vi "Unload Plugin.vi"(8 "error in (no error)":errorcluster, 10 "Unique Name":string, 11 "Launcher in":refnum<class "Plugin Manager.lvclass">) -> (0 "error out":errorcluster, 3 "Launcher out":refnum<class "Plugin Manager.lvclass">)   [LabVIEW 2021, in "Plugin Manager.lvclass"]
uses:
  Plugin Manager.lvclass
  Plugin Manager.lvclass/Plugin Manager.ctl
  CIFCore/Common/Typedef/Errors.ctl
  CIFCore/Common/Utilities/Append Error Location.vi
  CIFCore/Common/CIFCoreCommon.lvlib
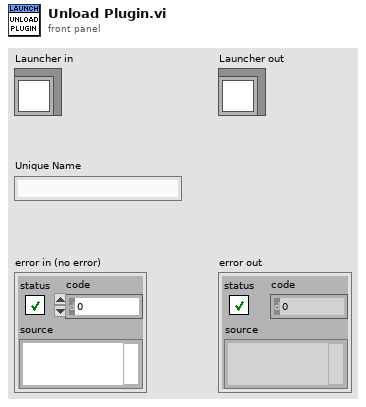
[diagram p1: front panel]
types:
  T1 = typedef "CIFCoreCommon.lvlib/Errors.ctl" = enum16{"Invalid Clock ID", "Long Sleep", "gRPC Server Not Found", "Config Parse", "Timestamp Wrap", "Delayed Execution", "Duplicate Channel", "Missing Channel", "Incorrect Type", "Flatten Error", "Unflatten Data", "Unique Name", "Plugin Not Found"}
  T2 = typedef "Plugin Manager.lvclass/Plugin Management Data.ctl" = cluster{"vi reference":refnum<vi>, "Plugin Type":string, "Unique Name":string, "Load Timestamp":u64, "gRPC Port":i32, "Version":T3}
  T3 = typedef "CIFCoreCommon.lvlib/Version.ctl" = cluster{"Major":i32, "Minor":i32, "Fix":i32, "Build":i32}
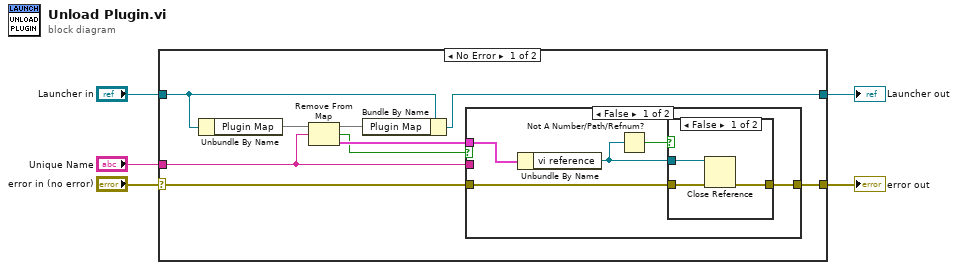
[diagram p0: block diagram]
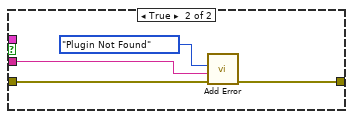
[diagram p3: hidden frame]
diagram:
  n1 = case shown="No Error" "error in (no error)" {
    selector: "error in (no error)" -> [w14 w29]
    tunnel: [w13 w29] -> w4
    tunnel: [w6 w28] -> w2
    tunnel: "Launcher in" -> [w8 w28]
    tunnel: "Unique Name" -> [w11 _]
    frame No Error {
      n2 = Unbundle By Name(w8) -> ("Plugin Map"=w12:map{string, T2})
      n3 = Remove From Map(10:w11, 11:w12) -> (1:w10:T2, 2:w9:bool, 3:w7:map{string, T2})
      n4 = Bundle By Name(cluster=w8, "Plugin Map"=w7) -> (w6:refnum<class "Plugin Manager.lvclass">)
      n5 = case shown="False" w9 {
        tunnel: w14 -> [w16 w27]
        tunnel: [w15 w24] -> w13
        tunnel: w11 -> [_ w25]
        tunnel: w10 -> [w19 _]
        frame False {
          n6 = Unbundle By Name(w19) -> ("vi reference"=w18:refnum<vi>)
          n7 = Not A Number/Path/Refnum?(number/path/refnum=w18) -> (NaN/Path/Refnum?=w17:bool)
          n8 = case shown="False" w17 {
            tunnel: w18 -> [w22 _]
            tunnel: w16 -> [w21 w23]
            tunnel: [w20 w23] -> w15
            frame False {
              n9 = Close Reference(reference=w22, error in (no error)=w21) -> (error out=w20:errorcluster)
            }
            frame True {
            }
          }
        }
        frame True {
          n10 = call "Add Error.vi"("error in (no error)"=w27, "String to Append"=w25, "Error"=Errors."Plugin Not Found") -> ("error out"=w24:errorcluster)  [unwired: 8 in]
        }
      }
    }
    frame Error {
    }
  }
  "error out" <- w4
  "Launcher out" <- w2
